vi "Subscribing Groups.vi"(8 "error in (no error)":errorcluster, 11 "SubscribedDataHandler in":refnum<class "SubscribedDataHandler.lvclass">) -> (0 "error out":errorcluster, 2 "Subscribing Groups":string[](array[string]))   [LabVIEW 2020, in "Vecto.lvlib" / "SubscribedDataHandler.lvclass"]
uses:
  SubscribedDataHandler.lvclass
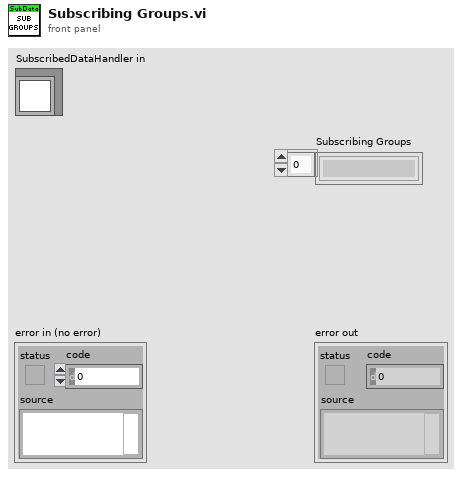
[diagram p1: front panel]
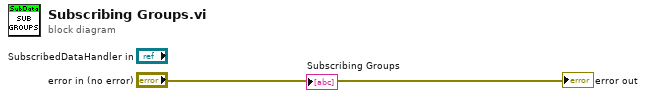
[diagram p0: block diagram]
diagram:
  "error out" <- "error in (no error)"
